vi "Test Tokenizer Implicit Commands.vi"(8 "error in (no error)":errorcluster) -> (0 "error out":errorcluster)   [LabVIEW 2019]
uses:
  PathTokenizer/PathTokenizer.lvclass
  PathTokenizer/PathTokenizer.lvclass/PathTokenizer.ctl
  <vilib>/addons/_JKI Toolkits/Caraya/classes/Assert/Assert Equal Value_Variant.vi
  <vilib>/addons/_JKI Toolkits/Caraya/classes/Test/Test.lvclass
  <vilib>/addons/_JKI Toolkits/Caraya/classes/Assert/Assert.lvclass
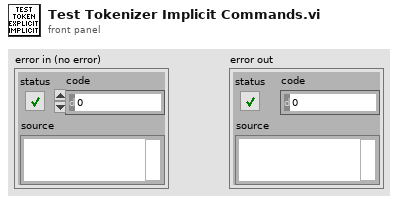
[diagram p1: front panel]
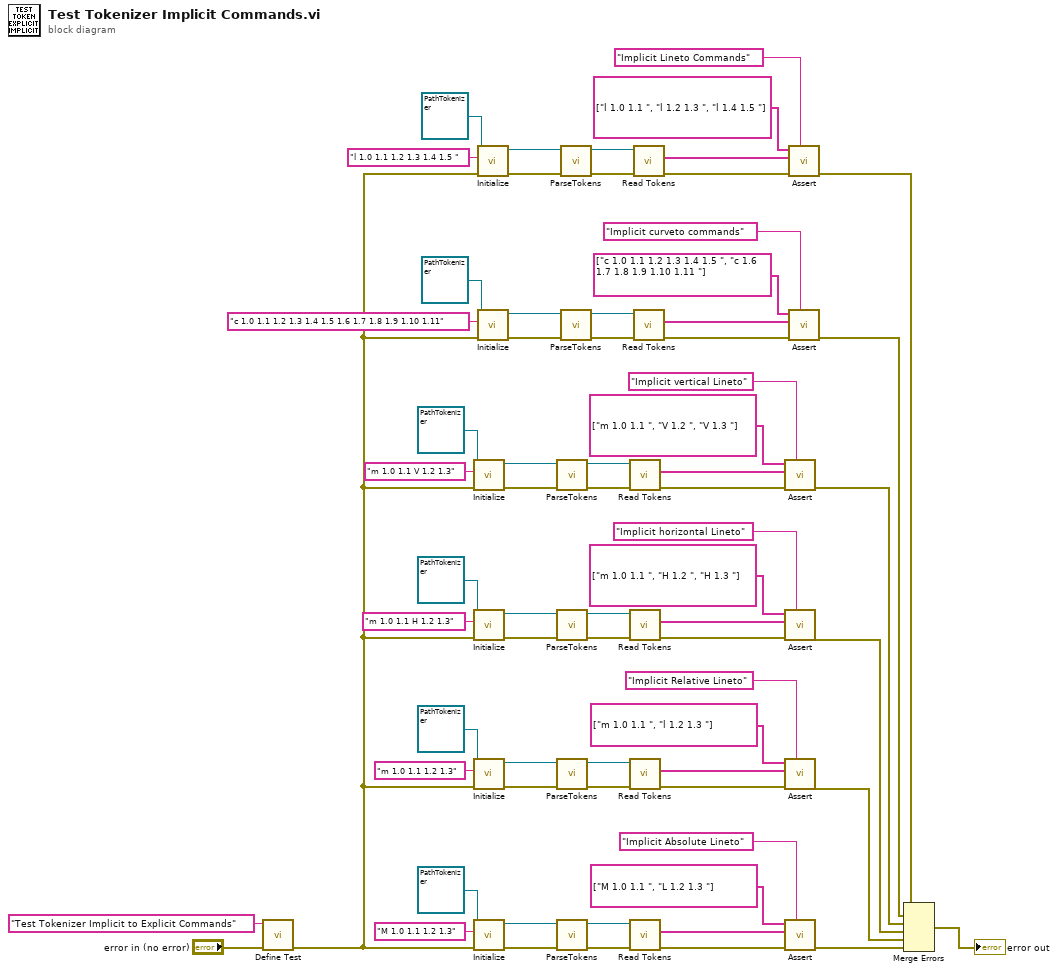
[diagram p0: block diagram]
diagram:
  n1 = call <vilib>:"Define Test.vi"("error in (no error)"="error in (no error)", "Label (VI Title)"="Test Tokenizer Implicit to Explicit Commands") -> ("error out"=w1:errorcluster)  [unwired: 8 in, 1 out]
  n2 = call "Initialize.vi"("error in (no error)"=w1, "Path Command Text"="m 1.0 1.1 V 1.2 1.3", "PathTokenizer in"=refnum<class "PathTokenizer.lvclass"> refnum) -> ("error out"=w33:errorcluster, "PathTokenizer out"=w32:refnum<class "PathTokenizer.lvclass">)  [unwired: 7 in]
  n3 = call "Initialize.vi"("error in (no error)"=w1, "Path Command Text"="m 1.0 1.1 H 1.2 1.3", "PathTokenizer in"=refnum<class "PathTokenizer.lvclass"> refnum) -> ("error out"=w37:errorcluster, "PathTokenizer out"=w38:refnum<class "PathTokenizer.lvclass">)  [unwired: 7 in]
  n4 = call "Initialize.vi"("error in (no error)"=w1, "Path Command Text"="m 1.0 1.1 1.2 1.3", "PathTokenizer in"=refnum<class "PathTokenizer.lvclass"> refnum) -> ("error out"=w55:errorcluster, "PathTokenizer out"=w54:refnum<class "PathTokenizer.lvclass">)  [unwired: 7 in]
  n5 = call "Initialize.vi"("error in (no error)"=w1, "Path Command Text"="M 1.0 1.1 1.2 1.3", "PathTokenizer in"=refnum<class "PathTokenizer.lvclass"> refnum) -> ("error out"=w59:errorcluster, "PathTokenizer out"=w60:refnum<class "PathTokenizer.lvclass">)  [unwired: 7 in]
  n6 = call "Initialize.vi"("error in (no error)"=w1, "Path Command Text"="l 1.0 1.1 1.2 1.3 1.4 1.5 ", "PathTokenizer in"=refnum<class "PathTokenizer.lvclass"> refnum) -> ("error out"=w10:errorcluster, "PathTokenizer out"=w9:refnum<class "PathTokenizer.lvclass">)  [unwired: 7 in]
  n7 = call "Initialize.vi"("error in (no error)"=w1, "Path Command Text"="c 1.0 1.1 1.2 1.3 1.4 1.5 1.6 1.7 1.8 1.9 1.10 1.11", "PathTokenizer in"=refnum<class "PathTokenizer.lvclass"> refnum) -> ("error out"=w16:errorcluster, "PathTokenizer out"=w17:refnum<class "PathTokenizer.lvclass">)  [unwired: 7 in]
  n8 = call "ParseTokens.vi"("error in (no error)"=w33, "PathTokenizer in"=w32) -> ("error out"=w28:errorcluster, "PathTokenizer out"=w29:refnum<class "PathTokenizer.lvclass">)  [unwired: 8 in]
  n9 = call "ParseTokens.vi"("error in (no error)"=w37, "PathTokenizer in"=w38) -> ("error out"=w42:errorcluster, "PathTokenizer out"=w41:refnum<class "PathTokenizer.lvclass">)  [unwired: 8 in]
  n10 = call "ParseTokens.vi"("error in (no error)"=w55, "PathTokenizer in"=w54) -> ("error out"=w50:errorcluster, "PathTokenizer out"=w51:refnum<class "PathTokenizer.lvclass">)  [unwired: 8 in]
  n11 = call "ParseTokens.vi"("error in (no error)"=w59, "PathTokenizer in"=w60) -> ("error out"=w64:errorcluster, "PathTokenizer out"=w63:refnum<class "PathTokenizer.lvclass">)  [unwired: 8 in]
  n12 = call "ParseTokens.vi"("error in (no error)"=w10, "PathTokenizer in"=w9) -> ("error out"=w5:errorcluster, "PathTokenizer out"=w6:refnum<class "PathTokenizer.lvclass">)  [unwired: 8 in]
  n13 = call "ParseTokens.vi"("error in (no error)"=w16, "PathTokenizer in"=w17) -> ("error out"=w21:errorcluster, "PathTokenizer out"=w20:refnum<class "PathTokenizer.lvclass">)  [unwired: 8 in]
  n14 = call "Read Tokens.vi"("error in (no error)"=w28, "PathTokenizer in"=w29) -> ("error out"=w25:errorcluster, "Tokens"=w27:string[])  [unwired: 7 in, 1 out]
  n15 = call "Read Tokens.vi"("error in (no error)"=w42, "PathTokenizer in"=w41) -> ("error out"=w45:errorcluster, "Tokens"=w43:string[])  [unwired: 7 in, 1 out]
  n16 = call "Read Tokens.vi"("error in (no error)"=w50, "PathTokenizer in"=w51) -> ("error out"=w47:errorcluster, "Tokens"=w49:string[])  [unwired: 7 in, 1 out]
  n17 = call "Read Tokens.vi"("error in (no error)"=w64, "PathTokenizer in"=w63) -> ("error out"=w67:errorcluster, "Tokens"=w65:string[])  [unwired: 7 in, 1 out]
  n18 = call "Read Tokens.vi"("error in (no error)"=w5, "PathTokenizer in"=w6) -> ("error out"=w3:errorcluster, "Tokens"=w4:string[])  [unwired: 7 in, 1 out]
  n19 = call "Read Tokens.vi"("error in (no error)"=w21, "PathTokenizer in"=w20) -> ("error out"=w23:errorcluster, "Tokens"=w22:string[])  [unwired: 7 in, 1 out]
  n20 = call-poly <vilib>:"Assert.vi"("Label"="Implicit vertical Lineto", "error in (no error)"=w25, "Y"=w27, "X"=string[] ["m 1.0 1.1 ", "V 1.2 ", "V 1.3 "] ("Tokens")) -> ("error out"=w24:errorcluster)  [unwired: 6 in, 1 out]
  n21 = call-poly <vilib>:"Assert.vi"("Label"="Implicit horizontal Lineto", "error in (no error)"=w45, "Y"=w43, "X"=string[] ["m 1.0 1.1 ", "H 1.2 ", "H 1.3 "] ("Tokens")) -> ("error out"=w35:errorcluster)  [unwired: 6 in, 1 out]
  n22 = call-poly <vilib>:"Assert.vi"("Label"="Implicit Relative Lineto", "error in (no error)"=w47, "Y"=w49, "X"=string[] ["m 1.0 1.1 ", "l 1.2 1.3 "] ("Tokens")) -> ("error out"=w46:errorcluster)  [unwired: 6 in, 1 out]
  n23 = call-poly <vilib>:"Assert.vi"("Label"="Implicit Absolute Lineto", "error in (no error)"=w67, "Y"=w65, "X"=string[] ["M 1.0 1.1 ", "L 1.2 1.3 "] ("Tokens")) -> ("error out"=w58:errorcluster)  [unwired: 6 in, 1 out]
  n24 = call-poly <vilib>:"Assert.vi"("Label"="Implicit Lineto Commands", "error in (no error)"=w3, "Y"=w4, "X"=string[] ["l 1.0 1.1 ", "l 1.2 1.3 ", "l 1.4 1.5 "] ("Tokens")) -> ("error out"=w2:errorcluster)  [unwired: 6 in, 1 out]
  n25 = call-poly <vilib>:"Assert.vi"("Label"="Implicit curveto commands", "error in (no error)"=w23, "Y"=w22, "X"=string[] ["c 1.0 1.1 1.2 1.3 1.4 1.5 ", "c 1.6 1.7 1.8 1.9 1.10 1.11 "] ("Tokens")) -> ("error out"=w14:errorcluster)  [unwired: 6 in, 1 out]
  n26 = Merge Errors(w2, w14, w24, w35, w46, w58) -> (→"error out":errorcluster)
